vi "Update Inited At.vi"(8 "error in (no error)":errorcluster, 10 "Inited At":string, 11 "Example View in":refnum<class "Example View Actor.lvclass">) -> (0 "error out":errorcluster, 3 "Example View out":refnum<class "Example View Actor.lvclass">)   [LabVIEW 2023, in "Example Event Actors.lvlib" / "Example View Actor.lvlib" / "Example View Actor.lvclass"]
uses:
  Example View Actor.lvclass
  Example View Actor.lvclass/Example View Actor.ctl
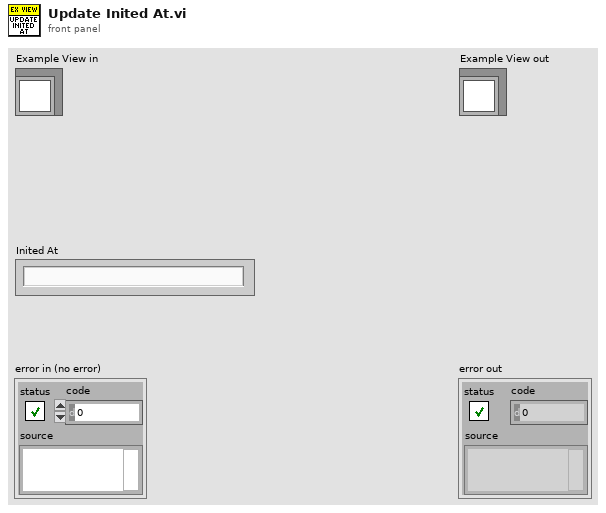
[diagram p1: front panel]
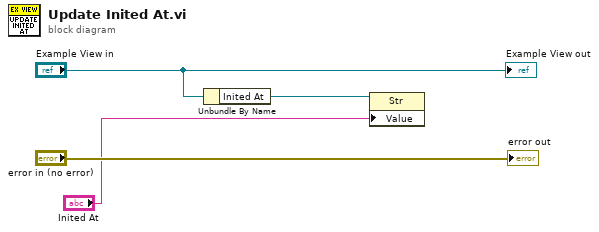
[diagram p0: block diagram]
diagram:
  n1 = Unbundle By Name("Example View in") -> ("Inited At"=w2:refnum<vi>)
  n2 = property class="Str"(reference=w2, "Value"="Inited At") -> ()  [unwired: 1 in, 2 out]
  "error out" <- "error in (no error)"
  "Example View out" <- "Example View in"
